vi "Chart - Load History.vi"(5 "time stamp":timestamp, 8 "Error In":errorcluster, 9 "Filestream":string, 10 "Load From File":bool=TRUE, 11 "file path (dialog if empty)":path=path "C:/Temp/SRTRS4070_Host/Data_Host/2014/08/0090300746_20140822_143302.dat") -> (0 "Error Out":errorcluster, 1 "Plot Names":string[](array[string]), 2 "t0 time stamp":timestamp, 3 "History":dynamicdata[](array[waveform]), 4 "size(s)":i32[](array[numeric]), 7 "all rows":dbl[][](array[numeric]))   [LabVIEW 2013]
panel:
  out "File Error":errorcluster
  out "File logging interval (minutes)":dbl
  in  "Update Chart":bool
  in  "Update Graph":bool
  out "Graph":cluster{"all rows":dbl[], "all rows":dbl[]}[](graph)
  out "element":i32
  out "# of channels":i32
  out "Transaction No":string
  out "Waveform Chart":dynamicdata(graph)
  # "From Calling VI"
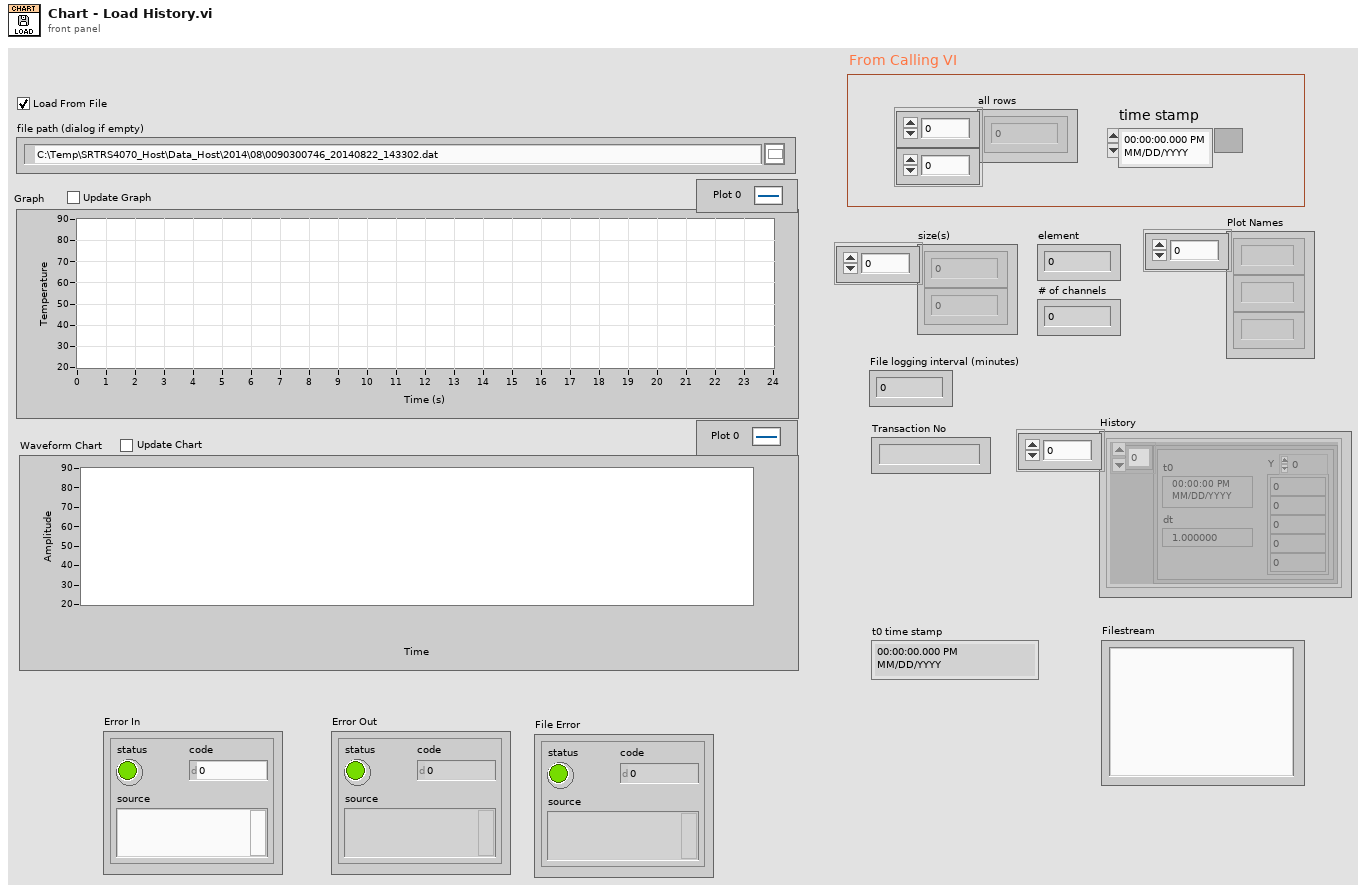
[diagram p1: front panel]
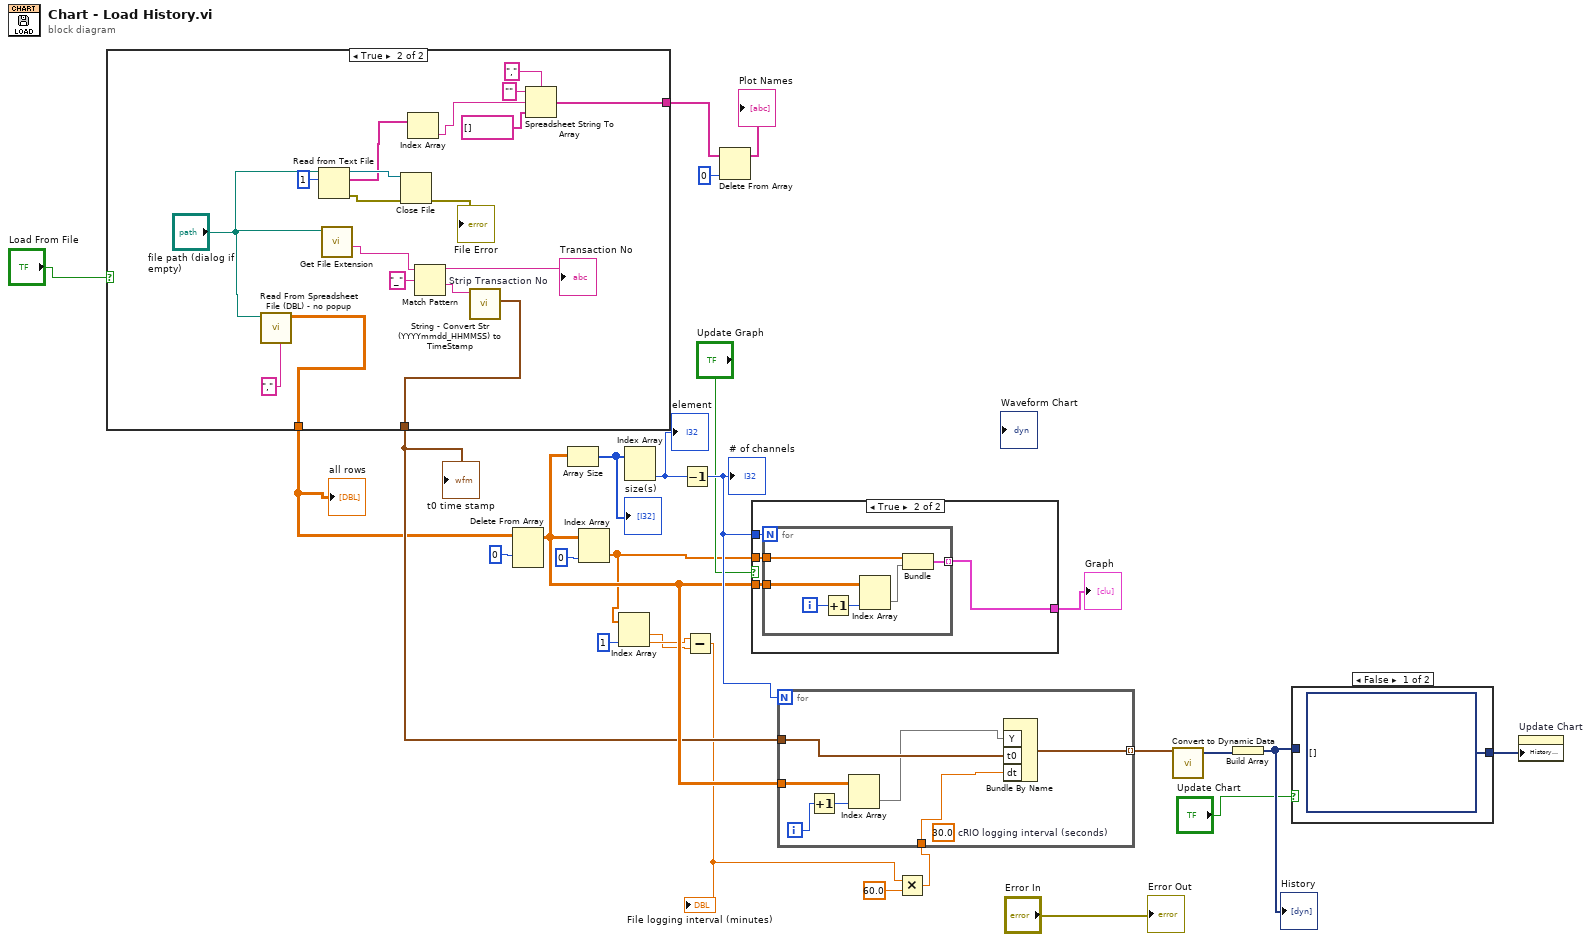
[diagram p0: block diagram]
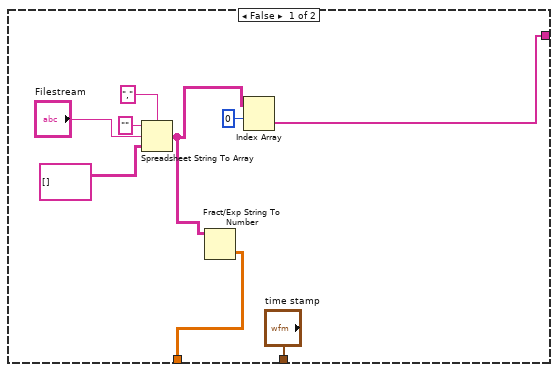
[diagram p2: hidden frame]
diagram:
  n1 = case shown="True" "Load From File" {
    tunnel: [w33 w37] -> w4
    tunnel: ["time stamp" w50] -> w13
    tunnel: [w30 w40] -> w1
    frame False {
      n2 = Spreadsheet String To Array(delimiter (Tab)=",", format string="", spreadsheet string="Filestream", array type (2D Dbl)=string[][] []) -> (array=w32:string[][])
      n3 = Fract/Exp String To Number(string=w32) -> (number=w33:dbl[][])  [unwired: 3 in, 1 out]
      n4 = Index Array(array=w32, index (row)=0) -> (element=w30:string[])  [unwired: 1 in]
    }
    frame True {
      n5 = call "Read From Spreadsheet File (DBL) - no popup.vi"("delimiter (\\t)"="," ("delimiter (\\t)"), "file path (dialog if empty)"="file path (dialog if empty)") -> ("all rows"=w37:dbl[][])  [unwired: 5 in, 4 out]
      n6 = Read from Text File(file (use dialog)="file path (dialog if empty)", count=1) -> (refnum out=w48:refnum<file>, text=w45:string[], error out=w47:errorcluster)  [unwired: 2 in, 1 out]
      n7 = call <vilib>:"Get File Extension.vi"("file"="file path (dialog if empty)") -> ("filename without extension"=w52:string)  [unwired: 7 in, 3 out]
      n8 = Close File(refnum=w48, error in=w47) -> (error out=→"File Error":errorcluster)  [unwired: 1 out]
      n9 = Index Array(array=w45) -> (element=w44:string)  [unwired: 1 in]
      n10 = Match Pattern "Strip Transaction No"(string=w52, regular expression="_") -> (before substring=→"Transaction No":string, after substring=w51:string)  [unwired: 1 in, 2 out]
      n11 = call "String - Convert Str (YYYYmmdd_HHMMSS) to TimeStamp.vi"("YYYYmmdd_HHMMSS"=w51) -> ("time stamp"=w50:timestamp)  [unwired: 8 in, 2 out]
      n12 = Spreadsheet String To Array(delimiter (Tab)=",", format string="", spreadsheet string=w44, array type (2D Dbl)=string[] []) -> (array=w40:string[])
    }
  }
  "t0 time stamp" <- w13
  "all rows" <- w4
  n13 = Delete From Array(array=w4, index (row)=0) -> (array with subset deleted=w22:dbl[][])  [unwired: 2 in, 1 out]
  n14 = Array Size(array=w22) -> (size(s)=w26:i32[])
  "size(s)" <- w26
  n15 = Index Array(array=w22, index (col)=0 ("disabled index (col)")) -> (element=w12:dbl[])  [unwired: 1 in]
  n16 = Index Array(array=w12, index #2=1 ("index")) -> (element #1=w9:dbl, element #2=w10:dbl)  [unwired: 1 in]
  n17 = Index Array(array=w26) -> (element #2=w27:i32)  [unwired: 2 in, 1 out]
  "element" <- w27
  n18 = Decrement(x=w27) -> (x-1=w23:i32)
  "# of channels" <- w23
  n19 = Subtract(x=w10, y=w9) -> (x-y=w8:dbl)
  "File logging interval (minutes)" <- w8
  n20 = Delete From Array(array=w1, index=0) -> (array with subset deleted=→"Plot Names":string[])  [unwired: 1 in, 1 out]
  n21 = case shown="True" "Update Graph" {
    tunnel: w12 -> [_ w58]
    tunnel: w23 -> [_ w57]
    tunnel: w22 -> [_ w56]
    tunnel: [_ w55] -> w16
    frame False {
    }
    frame True {
      n22 = for {
        N: w57 -> [_]
        tunnel: w56 -> [w64]
        tunnel: w58 -> [w61]
        tunnel: [w59] -> w55 mode=indexing
        i -> [w62]
        n23 = Increment(x=w62) -> (x+1=w63:i32)
        n24 = Index Array(array=w64, index (col)=w63) -> (element=w60:dbl[])  [unwired: 1 in]
        n25 = Bundle("all rows"=w61, "all rows"=w60) -> (w59:cluster{"all rows":dbl[], "all rows":dbl[]})  [unwired: 1 in]
      }
    }
  }
  "Graph" <- w16
  n26 = Multiply(x=w8, y=60.0) -> (x*y=w6:dbl)
  n27 = for {
    N: w23 -> [_]
    tunnel: [w71] -> w18 mode=indexing
    tunnel: w13 -> [w70]
    tunnel: w22 -> [w67]
    tunnel: w6 -> [w65]
    i -> [w69]
    (unwired) 30.0  # cRIO logging interval (seconds)
    n28 = Increment(x=w69) -> (x+1=w68:i32)
    n29 = Index Array(array=w67, index (col)=w68) -> (element=w66:dbl[])  [unwired: 1 in]
    n30 = Bundle By Name("Y"=w66, "t0"=w70, "dt"=w65) -> (w71:waveform(dbl))  [unwired: 1 in]
  }
  n31 = call "Convert to Dynamic Data"("Array of Waveforms"=w18) -> ("Dynamic Data Type"=w19:dynamicdata)  [unwired: 3 in]
  n32 = Build Array(w19) -> (w20:dynamicdata[])
  "History" <- w20
  n33 = case shown="False" "Update Chart" {
    tunnel: w20 -> [_ w73]
    tunnel: [dynamicdata[] [] w73] -> w15
    frame False {
    }
    frame True {
    }
  }
  n34 = property on="Update Chart" class="WFChart (strict)"("History Data"=w15) -> ()  [unwired: 2 in, 2 out]
  "Error Out" <- "Error In"
